vi "MVC OOP.vi"() -> ()   [LabVIEW 2011]
doc: "This VI is a function generator utilising a class."
uses:
  Controls/Command.ctl
  Class/Waveform.lvclass
panel:
  in  "FFT Signal":bool
  in  "Gen Signal":bool
  in  "Frequency":dbl(knob) scale=0.0..11.0
  out "Waveform Graph":waveform(dbl)(graph)
  in  "stop":bool
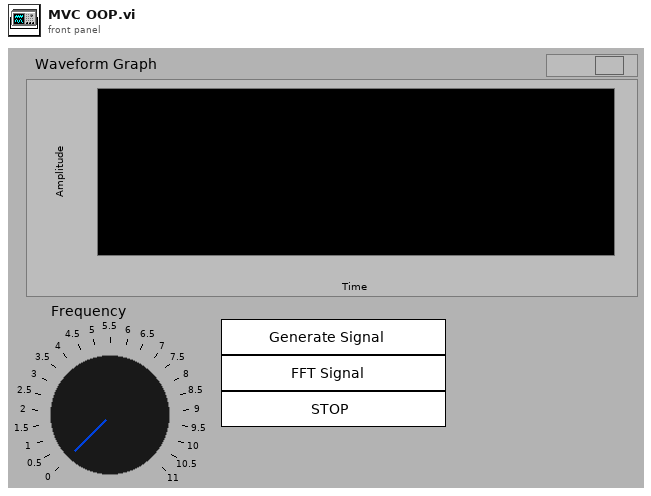
[diagram p1: front panel]
types:
  T1 = typedef "Command.ctl" = enum16{"Create Signal", "FFT Signal", "Set Frequency", "Stop", "Display", "Set Type"}
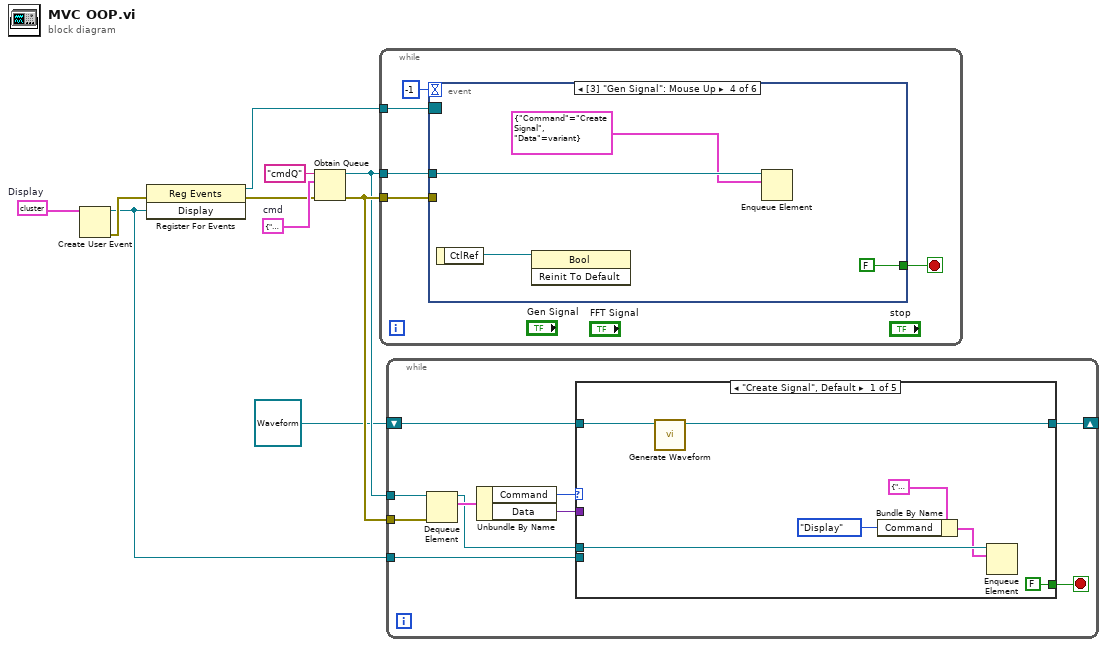
[diagram p0: block diagram]
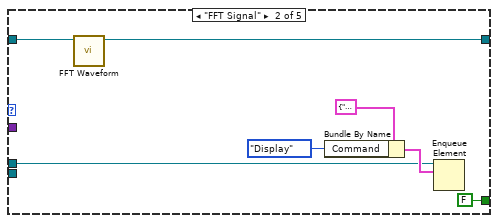
[diagram p2: hidden frame]
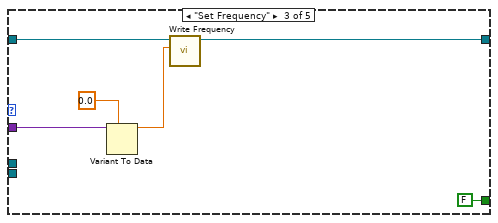
[diagram p3: hidden frame]
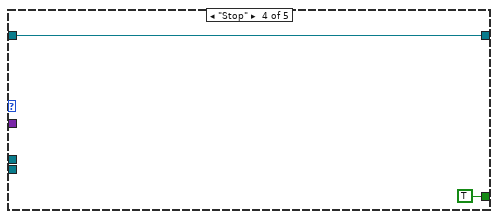
[diagram p4: hidden frame]
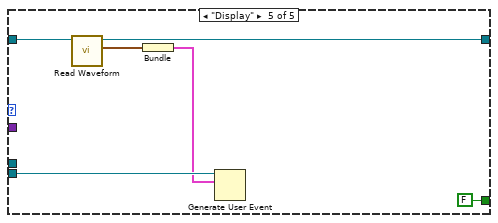
[diagram p5: hidden frame]
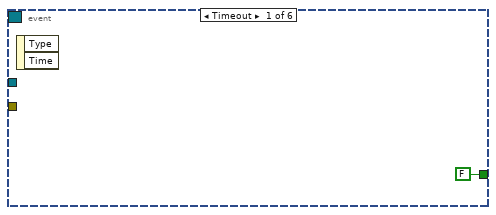
[diagram p6: hidden frame]
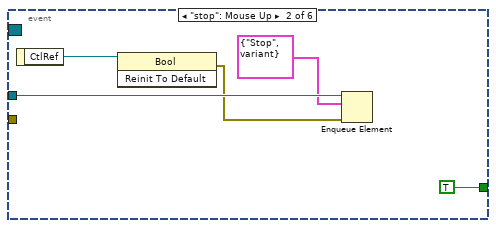
[diagram p7: hidden frame]
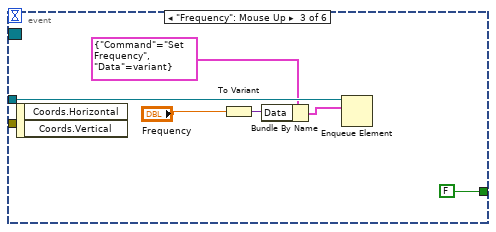
[diagram p8: hidden frame]
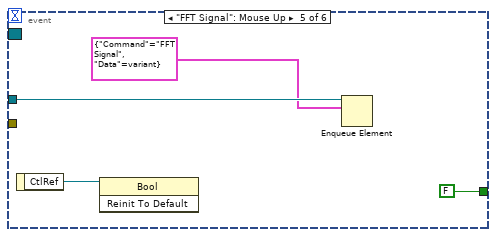
[diagram p9: hidden frame]
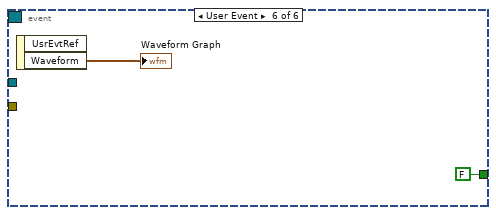
[diagram p10: hidden frame]
diagram:
  w7 = cluster{"Waveform":waveform(dbl)} {"Waveform"={"t0"=timestamp(0 s since 1904-01-01), "dt"=1.0, "Y"=[]}}  # Display
  w10 = cluster{"Command":T1, "Data":variant} {"Command"=enum."Create Signal", "Data"=variant}  # cmd
  n1 = Create User Event(user event datatype=w7) -> (user event=w2:refnum<user-event>, error out=w6:errorcluster)  [unwired: 1 in]
  n2 = register-events(error in=w6, w2) -> (reference out=w5:refnum<event-registration>, error out=w8:errorcluster)  [unwired: 1 in]
  n3 = Obtain Queue(name (unnamed)="cmdQ", element data type=w10, error in (no error)=w8) -> (queue out=w3:refnum<queue>, error out=w4:errorcluster)  [unwired: 2 in, 1 out]
  n4 = while {
    tunnel: w3 -> [w14]
    tunnel: w5 -> [w12]
    tunnel: w4 -> [w11]
    stop <- w13 stop-if-true
    n5 = event shown="[3] \"Gen Signal\": Mouse Up" {
      selector: w12 -> [_ _ _ _ _ _]
      dyn-events: _ -> [_ _ _ _ _ _]
      timeout: -1 -> [_ _ _ _ _ _]
      tunnel: w14 -> [_ w20 w27 w31 w35 _]
      tunnel: [FALSE TRUE FALSE FALSE FALSE FALSE] -> w13
      tunnel: w11 -> [_ _ _ _ _ _]
      event Timeout {
        n6 = event-data() -> ()  [unwired: 1 in, 2 out]
      }
      event "stop": Mouse Up {
        n7 = event-data() -> ("CtlRef"=w21:refnum<vi>)  [unwired: 1 in]
        n8 = invoke class="Bool" method="Reinit To Default"(reference=w21) -> (error out=w19:errorcluster)  [unwired: 2 in, 2 out]
        n9 = Enqueue Element(queue=w20, element=cluster{"Command":T1, "Data":variant} {"Command"=enum."Stop", "Data"=variant}, error in (no error)=w19) -> ()  [unwired: 1 in, 3 out]
      }
      event "Frequency": Mouse Up {
        n10 = event-data() -> ()  [unwired: 1 in, 2 out]
        n11 = To Variant(anything="Frequency") -> (Variant=w23:variant)
        n12 = Bundle By Name(cluster=cluster{"Command":T1, "Data":variant} {"Command"=enum."Set Frequency", "Data"=variant} ("element"), "Data"=w23) -> (w24:cluster{"Command":T1, "Data":variant})
        n13 = Enqueue Element(queue=w27, element=w24) -> ()  [unwired: 2 in, 3 out]
      }
      event "Gen Signal": Mouse Up {
        n14 = event-data() -> ("CtlRef"=w28:refnum<vi>)  [unwired: 1 in]
        n15 = invoke class="Bool" method="Reinit To Default"(reference=w28) -> ()  [unwired: 2 in, 3 out]
        n16 = Enqueue Element(queue=w31, element=cluster{"Command":T1, "Data":variant} {"Command"=enum."Create Signal", "Data"=variant}) -> ()  [unwired: 2 in, 3 out]
      }
      event "FFT Signal": Mouse Up {
        n17 = event-data() -> ("CtlRef"=w32:refnum<vi>)  [unwired: 1 in]
        n18 = invoke class="Bool" method="Reinit To Default"(reference=w32) -> ()  [unwired: 2 in, 3 out]
        n19 = Enqueue Element(queue=w35, element=cluster{"Command":T1, "Data":variant} {"Command"=enum."FFT Signal", "Data"=variant}) -> ()  [unwired: 2 in, 3 out]
      }
      event User Event {
        n20 = event-data() -> ("Waveform"=→"Waveform Graph":waveform(dbl))  [unwired: 1 in, 1 out]
      }
    }
  }
  n21 = while {
    tunnel: w4 -> [w46]
    tunnel: w3 -> [w47]
    tunnel: w2 -> [w40]
    shift-right: [w38] -> _
    shift-left: refnum<class "Waveform.lvclass"> refnum ("Waveform.lvclass") -> [w39]
    stop <- w42 stop-if-true
    n22 = Dequeue Element(queue=w47, error in (no error)=w46) -> (queue out=w41:refnum<queue>, element=w45:cluster{"Command":T1, "Data":variant})  [unwired: 1 in, 2 out]
    n23 = Unbundle By Name(w45) -> ("Command"=w44:T1, "Data"=w43:variant)
    n24 = case shown="\"Create Signal\", Default" w44 {
      tunnel: w43 -> [_ _ w67 _ _]
      tunnel: [FALSE FALSE FALSE TRUE FALSE] -> w42
      tunnel: w41 -> [w54 w58 _ _ _]
      tunnel: w40 -> [_ _ _ _ w75]
      tunnel: w39 -> [w49 w56 w65 w68 w72]
      tunnel: [w48 w55 w62 w68 w70] -> w38
      frame "Create Signal", Default {
        n25 = call-dynamic "Generate Waveform.vi"("Waveform in"=w49) -> ("Waveform out"=w48:refnum<class "Waveform.lvclass">)  [unwired: 9 in, 1 out]
        n26 = Bundle By Name(cluster=cluster{"Command":T1, "Data":variant} {"Command"=enum."Create Signal", "Data"=variant} ("element"), "Command"=Command."Display") -> (w51:cluster{"Command":T1, "Data":variant})
        n27 = Enqueue Element(queue=w54, element=w51) -> ()  [unwired: 2 in, 3 out]
      }
      frame "FFT Signal" {
        n28 = call-dynamic "FFT Waveform.vi"("Waveform in"=w56) -> ("Waveform out"=w55:refnum<class "Waveform.lvclass">)  [unwired: 9 in, 1 out]
        n29 = Bundle By Name(cluster=cluster{"Command":T1, "Data":variant} {"Command"=enum."Create Signal", "Data"=variant} ("element"), "Command"=Command."Display") -> (w59:cluster{"Command":T1, "Data":variant})
        n30 = Enqueue Element(queue=w58, element=w59) -> ()  [unwired: 2 in, 3 out]
      }
      frame "Set Frequency" {
        n31 = Variant To Data(type=0.0 ("Frequency"), Variant=w67) -> (data=w63:dbl)  [unwired: 1 in, 1 out]
        n32 = call-dynamic "Write Frequency.vi"("Frequency"=w63, "Waveform in"=w65) -> ("Waveform out"=w62:refnum<class "Waveform.lvclass">)  [unwired: 8 in, 1 out]
      }
      frame "Stop" {
      }
      frame "Display" {
        n33 = call-dynamic "Read Waveform.vi"("Waveform in"=w72) -> ("Waveform"=w71:waveform(dbl), "Waveform out"=w70:refnum<class "Waveform.lvclass">)  [unwired: 8 in, 1 out]
        n34 = Bundle("Waveform"=w71) -> (w74:cluster{"Waveform":waveform(dbl)})  [unwired: 1 in]
        n35 = Generate User Event(user event=w75, event data cluster=w74) -> ()  [unwired: 1 in, 2 out]
      }
    }
  }
